vi "compare channel list to typedefs.vi"(8 "error in":errorcluster, 11 "fixed channel configuration":refnum<class "control module configuration.lvclass">) -> (0 "error out":errorcluster)   [LabVIEW 2013, in "control module configuration.lvclass"]
uses:
  control module configuration.lvclass
  control module configuration.lvclass/control module configuration.ctl
  <vilib>/NI/Tag Bus/tag/tag descriptor.lvclass/tag descriptor.ctl
  <vilib>/NI/Tag Bus Module Framework/channel/TBM channel.lvclass/TBM channel.ctl
  <vilib>/NI/Tag Bus/tag/read data type.vi
  <vilib>/NI/Tag Bus Module Framework/channel/Read channel classification.vi
  <vilib>/NI/Tag Bus/tag/read tag name.vi
  <vilib>/NI/Tag Bus/tag/tag descriptor.lvclass
  <vilib>/NI/Tag Bus Module Framework/channel/TBM channel.lvclass
  <vilib>/NI/Configuration Framework/NISE_CEF_TreeControl.lvlib
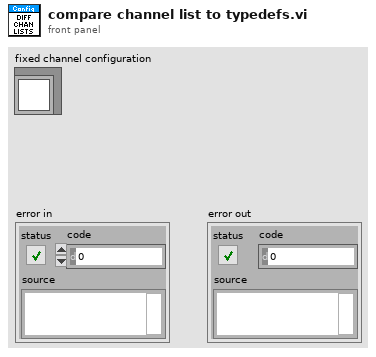
[diagram p1: front panel]
types:
  T1 = typedef "tag bus.lvlib/tag descriptor.lvclass/Data Type.ctl" = enum16{"Double", "Single", "I64", "I32", "I16", "I8", "U64", "U32", "U16", "U8", "Boolean", "String", "Array of Double", "Array of Single", "Array of I64", "Array of I32", "Array of I16", "Array of I8", "Array of U64", "Array of U32", "Array of U16", "Array of U8", "Array of Boolean", "Array of String"}
  T2 = typedef "TBM channel.lvclass/channel classification.ctl" = enum16{"input data", "output data", "processing parameter", "processing result"}
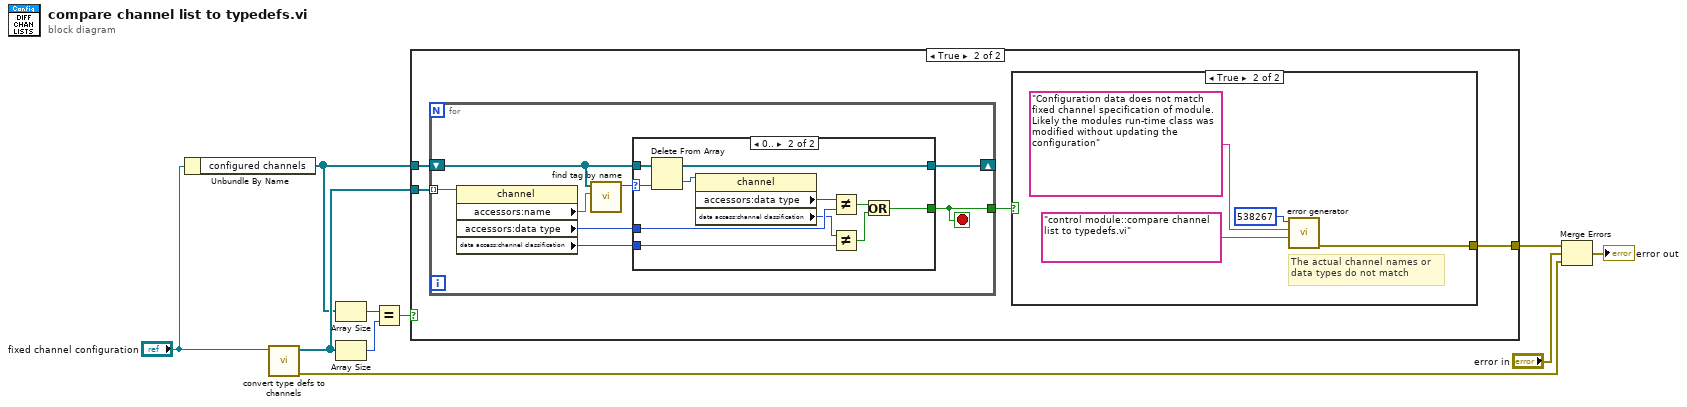
[diagram p0: block diagram]
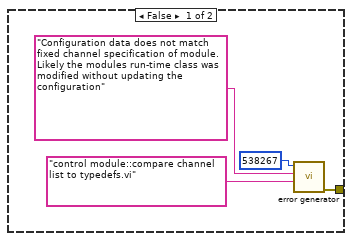
[diagram p2: hidden frame]
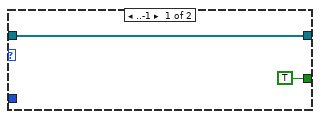
[diagram p3: hidden frame]
diagram:
  n1 = Unbundle By Name("fixed channel configuration") -> ("configured channels"=w1:refnum<class "TBM channel.lvclass">[])
  n2 = call "convert type defs to channels.vi"("fixed channel configuration"="fixed channel configuration") -> ("error out"=w3:errorcluster, "Array out"=w4:refnum<class "TBM channel.lvclass">[])  [unwired: 9 in]
  n3 = Array Size(array=w1) -> (size(s)=w8:i32)
  n4 = Array Size(array=w4) -> (size(s)=w9:i32)
  n5 = Equal?(x=w8, y=w9) -> (x = y?=w7:bool)
  n6 = case shown="True" w7 {
    tunnel: w1 -> [_ w17]
    tunnel: [w11 w18] -> w10
    tunnel: w4 -> [_ w16]
    frame False {
      n7 = call <vilib>:"error generator.vi"("source"="control module::compare channel list to typedefs.vi", "append error message"="Configuration data does not match fixed channel specification of module.  Likely the modules run-time class was modified without updating the configuration" ("source"), "error code (0)"=538267) -> ("error out"=w11:errorcluster)  [unwired: 6 in]
    }
    frame True {
      n8 = for {
        shift-right: [w23] -> _
        shift-left: w17 -> [w22]
        tunnel: w16 -> [w26] mode=indexing
        tunnel: [w19] -> w15
        stop <- w19 stop-if-true
        n9 = property class="channel"(reference=w26) -> ("accessors:name"=w25:string, "accessors:data type"=w21:T1, "data access:channel classification"=w20:T2)  [unwired: 1 in, 2 out]
        n10 = call <vilib>:"find tag by name.vi"("name"=w25, "tags in"=w22) -> ("index"=w24:i32)  [unwired: 9 in]
        n11 = case shown="0.." w24 {
          selector: w24 -> [_ w38]
          tunnel: [w28 w37] -> w23
          tunnel: w22 -> [w28 w39]
          tunnel: [TRUE w35] -> w19
          tunnel: w21 -> [_ w33]
          tunnel: w20 -> [_ w31]
          frame ..-1 {
          }
          frame 0.. {
            n12 = Delete From Array(array=w39, index=w38) -> (deleted portion=w36:refnum<class "TBM channel.lvclass">, array with subset deleted=w37:refnum<class "TBM channel.lvclass">[])  [unwired: 1 in]
            n13 = property class="channel"(reference=w36) -> ("accessors:data type"=w34:T1, "data access:channel classification"=w32:T2)  [unwired: 1 in, 2 out]
            n14 = Not Equal?(x=w34, y=w33) -> (x != y?=w29:bool)
            n15 = Not Equal?(x=w32, y=w31) -> (x != y?=w30:bool)
            n16 = Or(x=w29, y=w30) -> (x .or. y?=w35:bool)
          }
        }
      }
      n17 = case shown="True" w15 {
        tunnel: [_ w43] -> w18
        frame False {
        }
        frame True {
          # "The actual channel names or\ndata types do not match"
          n18 = call <vilib>:"error generator.vi"("source"="control module::compare channel list to typedefs.vi", "append error message"="Configuration data does not match fixed channel specification of module.  Likely the modules run-time class was modified without updating the configuration" ("source"), "error code (0)"=538267) -> ("error out"=w43:errorcluster)  [unwired: 6 in]
        }
      }
    }
  }
  n19 = Merge Errors(w10, "error in", w3) -> (→"error out":errorcluster)
